vi "RunScript.vi"(8 "error in (no error)":errorcluster, 9 "In":cluster{"X":dbl[][], "y":dbl[], "groups":dbl[]}={"X"=[[1.0, 2.0], [3.0, 4.0], [5.0, 6.0], [7.0, 8.0]], "y"=[1.0, 2.0, 3.0, 4.0], "groups"=[]}, 10 "function name":string="exec_code", 11 "Splitter in":refnum<class "Splitter.lvclass">) -> (0 "error out":errorcluster, 2 "Out":string, 3 "Splitter out":refnum<class "Splitter.lvclass">)   [LabVIEW 2020, in "Splitter.lvclass"]
uses:
  Splitter.lvclass
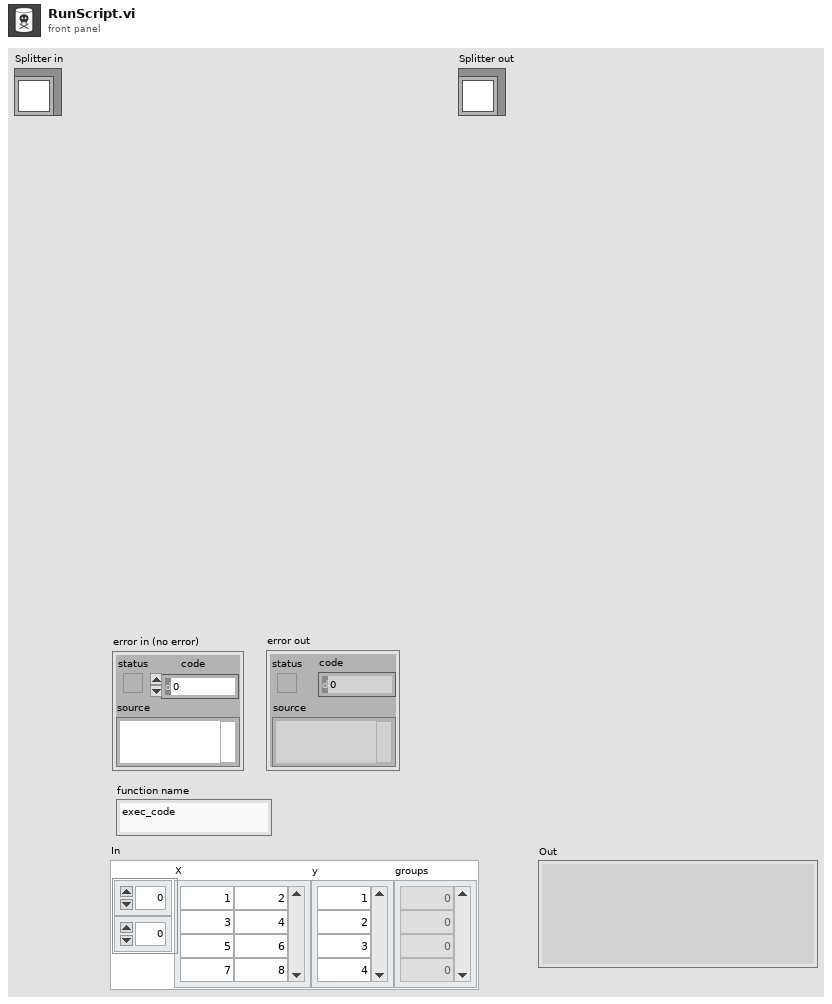
[diagram p1: front panel]
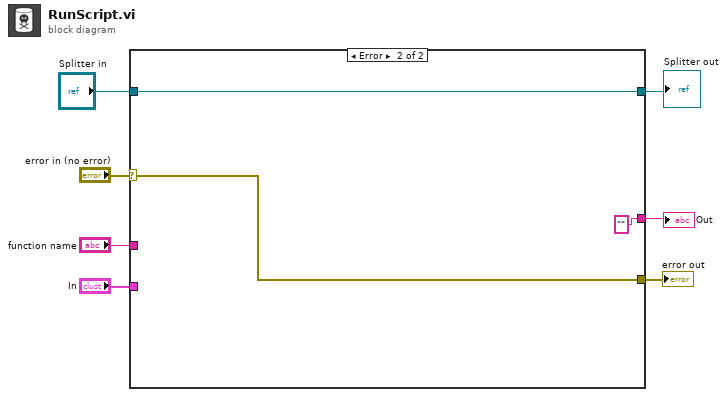
[diagram p0: block diagram]
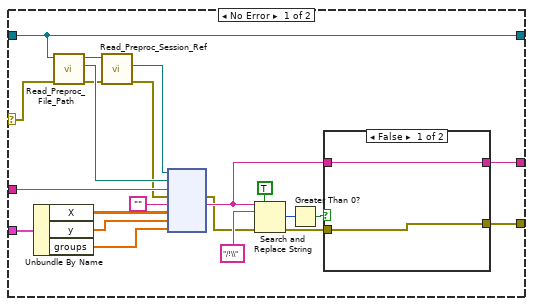
[diagram p2: hidden frame]
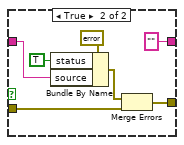
[diagram p3: hidden frame]
diagram:
  n1 = case shown="Error" "error in (no error)" {
    selector: "error in (no error)" -> [w14 w41]
    tunnel: [w21 w41] -> w6
    tunnel: "function name" -> [w29 _]
    tunnel: [w22 ""] -> w4
    tunnel: "Splitter in" -> [w16 w39]
    tunnel: [w16 w39] -> w2
    tunnel: "In" -> [w11 _]
    frame No Error {
      n2 = Unbundle By Name(w11) -> ("X"=w10:dbl[][], "y"=w9:dbl[], "groups"=w8:dbl[])
      n3 = call-dynamic "Read_Preproc_File_Path.vi"("error in (no error)"=w14, "Python in"=w16) -> ("error out"=w13:errorcluster, "File_Path"=w17:path, "Python out"=w15:refnum<class "Splitter.lvclass">)  [unwired: 7 in]
      n4 = call-dynamic "Read_Preproc_Session_Ref.vi"("error in (no error)"=w13, "Python in"=w15) -> ("error out"=w12:errorcluster, "Session_ref"=w18:refnum<k35>)  [unwired: 7 in, 1 out]
      n5 = node(w18, w17, w29, w12, "", w10, w9, w8) -> (w20:errorcluster, w23:string)  [unwired: 3 in, 3 out]
      n6 = Search and Replace String(replace all?=TRUE ("replace all? (F)"), input string=w23, search string="/!\\", error in=w20) -> (number of replacements=w27:i32, error out=w28:errorcluster)  [unwired: 4 in, 2 out]
      n7 = Greater Than 0?(x=w27) -> (x > 0?=w26:bool)
      n8 = case shown="False" w26 {
        tunnel: w28 -> [w30 w35]
        tunnel: [w30 w34] -> w21
        tunnel: w23 -> [w31 w32]
        tunnel: [w31 ""] -> w22
        frame False {
        }
        frame True {
          n9 = Bundle By Name(cluster=errorcluster {"status"=FALSE, "code"=0, "source"=""} ("error constant"), "status"=TRUE, "source"=w32) -> (w36:errorcluster)
          n10 = Merge Errors(w36, w35) -> (w34:errorcluster)
        }
      }
    }
    frame Error {
    }
  }
  "Splitter out" <- w2
  "error out" <- w6
  "Out" <- w4
